vi "get Free Running.vi"(11 "Clock Generator in":refnum<class "Clock Generator.lvclass">) -> (3 "Free Running":bool)   [LabVIEW 2021, in "Clock Generator.lvclass"]
uses:
  Clock Generator.lvclass
  Clock Generator.lvclass/Clock Generator.ctl
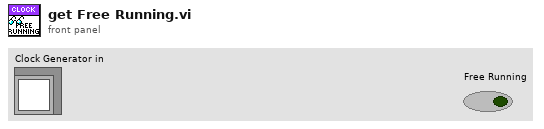
[diagram p1: front panel]
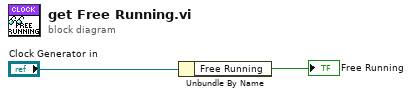
[diagram p0: block diagram]
diagram:
  n1 = Unbundle By Name("Clock Generator in") -> ("Free Running"=→"Free Running":bool)
